vi "Pusher_Client_Open.vi"(8 "ErrIn":errorcluster, 11 "api_key":string) -> (0 "ErrOut":errorcluster, 3 "Client out":refnum<class "Client.lvclass">)   [LabVIEW 2009, in "Client.lvclass"]
uses:
  Client.lvclass
  Client.lvclass/Client.ctl
panel:
  out "Reply":string
  in  "Client in":refnum<class "Client.lvclass">
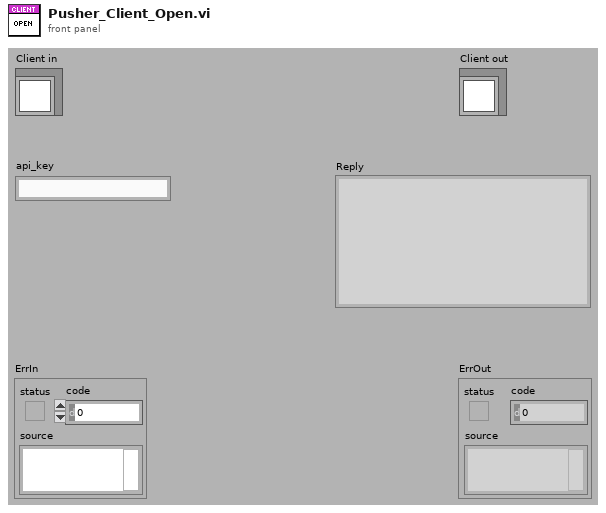
[diagram p1: front panel]
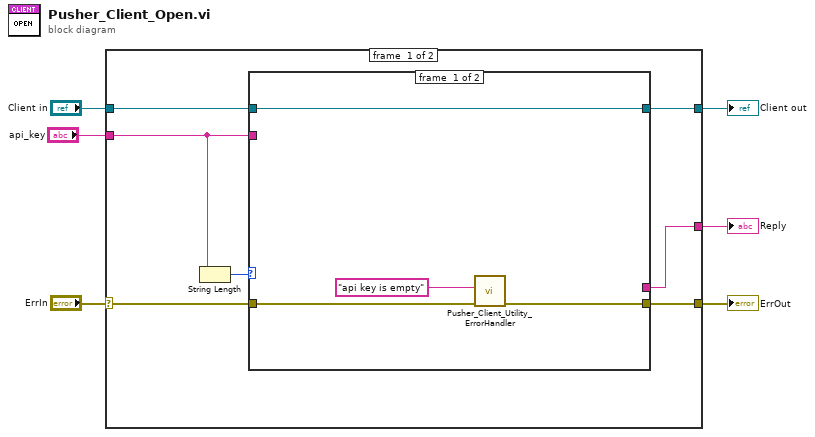
[diagram p0: block diagram]
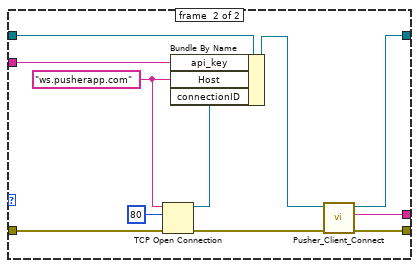
[diagram p2: hidden frame]
diagram:
  n1 = case shown="No Error" "ErrIn" {
    selector: "ErrIn" -> [w13 w30]
    tunnel: [w10 w30] -> w5
    tunnel: [w9 w29] -> w3
    tunnel: "Client in" -> [w12 w29]
    tunnel: "api_key" -> [w7 _]
    tunnel: [w11 _] -> w1
    frame #0 {
      n2 = String Length(string=w7) -> (length=w8:i32)
      n3 = case shown="1, Default" w8 {
        tunnel: w13 -> [w16 w28]
        tunnel: w12 -> [w17 w27]
        tunnel: w7 -> [_ w24]
        tunnel: [_ w20] -> w11
        tunnel: [w15 w19] -> w10
        tunnel: [w17 w18] -> w9
        frame #0 {
          n4 = call "Pusher_Client_Utility_ErrorHandler.vi"("ErrIn"=w16, "Additional Message"="api key is empty") -> ("ErrOut"=w15:errorcluster)  [unwired: 9 in]
        }
        frame #1 {
          w26 = "ws.pusherapp.com" ("Host")
          n5 = TCP Open Connection(address=w26, remote port or service name=u16 80, error in (no error)=w28) -> (connection ID=w23:refnum<k5>, error out=w21:errorcluster)  [unwired: 2 in]
          n6 = Bundle By Name(cluster=w27, "api_key"=w24, "Host"=w26, "connectionID"=w23) -> (w22:refnum<class "Client.lvclass">)
          n7 = call "Pusher_Client_Connect.vi"("ErrIn"=w21, "Client in"=w22) -> ("ErrOut"=w19:errorcluster, "Reply"=w20:string, "Client out"=w18:refnum<class "Client.lvclass">)  [unwired: 7 in]
        }
      }
    }
    frame #1 {
    }
  }
  "ErrOut" <- w5
  "Client out" <- w3
  "Reply" <- w1
